vi "Sub VI example 2.vi"() -> ()   [LabVIEW 2024]
panel:
  in  "Name 3":string
  in  "Switch 2":bool
  in  "X 3":dbl
  in  "Array 2":dbl[][](array[numeric])
  out "output cluster 2":T1
  out "output cluster":T1
  in  "Name 2":string
  out "Array":dbl[][](array[numeric])
  out "Name":string
  out "Switch":bool
  out "X 2":dbl
  out "X":dbl
  out "Cluster 2":T2
  in  "Cluster":T1
  out "I_ph":dbl
  in  "G (w/m^2)":dbl
  in  "T (K)":dbl
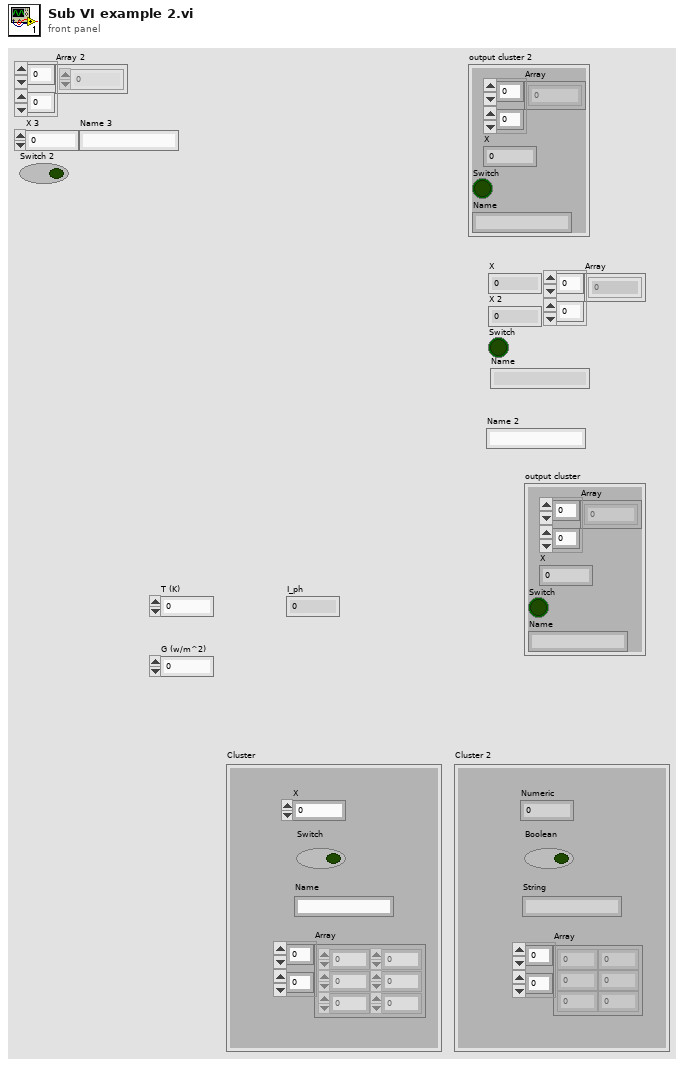
[diagram p1: front panel]
types:
  T1 = cluster{"Array":dbl[][], "X":dbl, "Switch":bool, "Name":string}
  T2 = cluster{"Array":dbl[][], "Numeric":dbl, "Boolean":bool, "String":string}
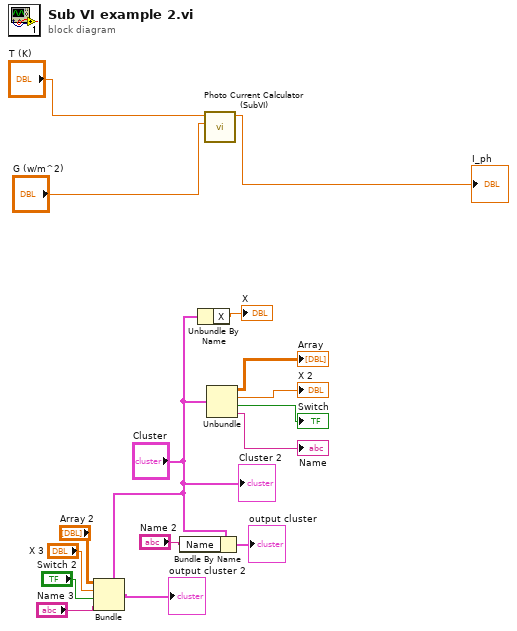
[diagram p0: block diagram]
diagram:
  n1 = Bundle(cluster="Cluster", "Array"="Array 2", "X"="X 3", "Switch"="Switch 2", "Name"="Name 3") -> (→"output cluster 2":T1)
  n2 = Bundle By Name(cluster="Cluster", "Name"="Name 2") -> (→"output cluster":T1)
  n3 = Unbundle By Name("Cluster") -> ("X"=→"X":dbl)
  n4 = call "Photo Current Calculator (SubVI).vi"("G (w/m^2)"="G (w/m^2)", "T (K)"="T (K)") -> ("I_ph"=→"I_ph":dbl)  [unwired: 9 in]
  n5 = Unbundle("Cluster") -> ("Array"=→"Array":dbl[][], "X"=→"X 2":dbl, "Switch"=→"Switch":bool, "Name"=→"Name":string)
  "Cluster 2" <- "Cluster"
